vi "XYStage.TestLauncher.vi"() -> ()   [LabVIEW 2013]
doc: "JKI State Machine Objects (SMO) 1.0.0.5\nJKI - JKI\nCopyright (c) 2016, JKI"
uses:
  <vilib>/JKI/JKI SMO/SMO/SMO.lvclass
  XYStage.lvclass
  <vilib>/JKI/JKI SMO/SMO/Typedefs/SMOState --Enum.ctl
  Typedefs/(real)Coords--Cluster.ctl
  Typedefs/Configuration--Cluster.ctl
  XYStage.Simulated/XYStage.Simulated.lvclass
  Typedefs/(counts)Coords--Cluster.ctl
panel:
  in  "Home":bool
  out "Move Complete":bool
  out "Counts":T1
  in  "List Positions":bool
  in  "Move to Position":bool
  in  "Named Positions":i32(listbox)
  in  "Name":string
  in  "Store Position":bool
  out "Current Position":T2
  in  "MoveRel":bool
  in  "Coords":T2
  in  "MoveAbs":bool
  out "error out":errorcluster
  in  "Stop":bool
  # "XY Stage Test Launcher"
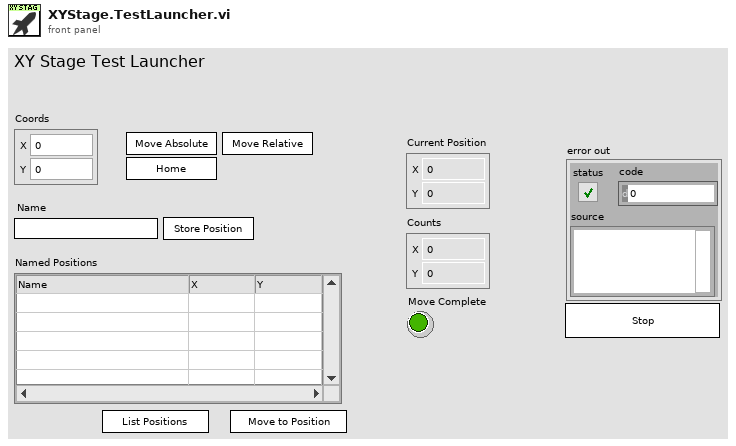
[diagram p1: front panel]
types:
  T1 = typedef "XYStage.lvclass/(counts)Coords--Cluster.ctl" = cluster{"X":i32, "Y":i32}
  T2 = typedef "XYStage.lvclass/(real)Coords--Cluster.ctl" = cluster{"X":dbl, "Y":dbl}
  T3 = typedef "XYStage.lvclass/Configuration--Cluster.ctl" = cluster{"Real-World Units":string, "Counts per Unit":dbl}
  T4 = typedef "SMO.lvclass/Public Events.ctl" = cluster{"Error":refnum<user-event>, "State":refnum<user-event>}
  T5 = typedef "XYStage.lvclass/PublicEvents--Cluster.ctl" = cluster{"MoveComplete":refnum<user-event>, "NewPosition":refnum<user-event>, "UpdatedNamedPosition":refnum<user-event>, "MoveStarted":refnum<user-event>}
  T6 = cluster{"Event Registration Refnum":refnum<event-registration>}
  T7 = typedef "SMO.lvclass/SMOState --Enum.ctl" = enum16{"unknown", "Created", "Started", "Stopped"}
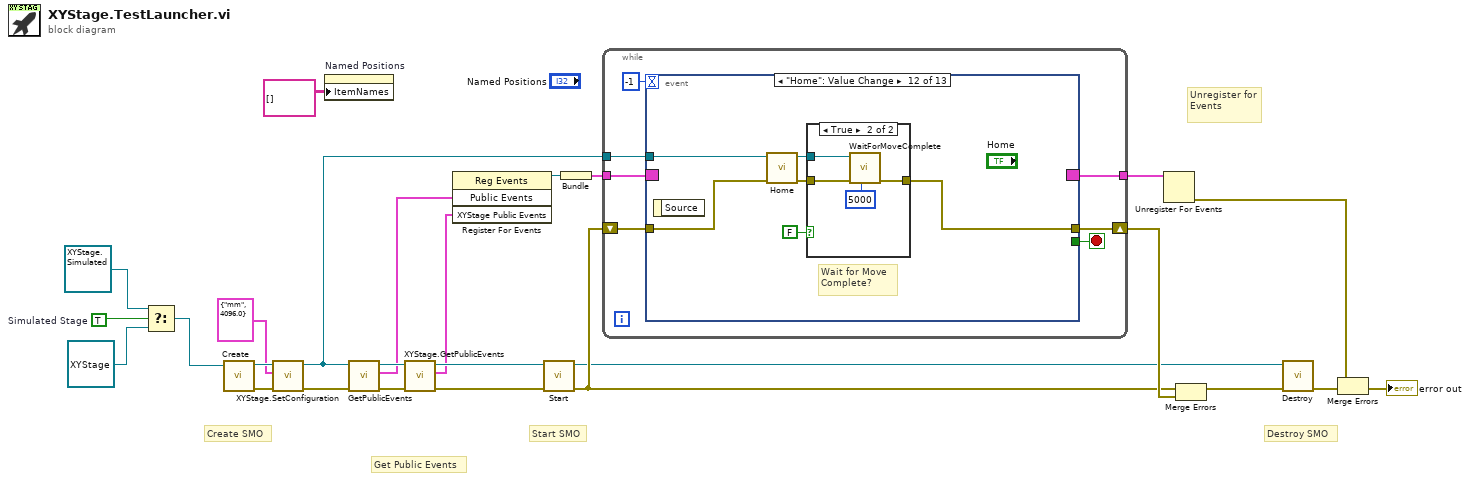
[diagram p0: block diagram]
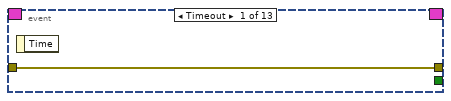
[diagram p2: hidden frame]
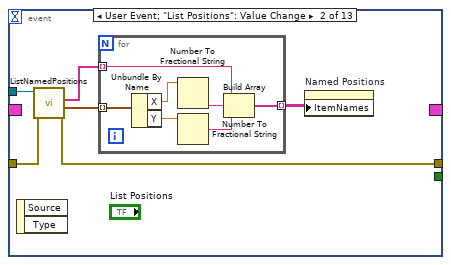
[diagram p3: hidden frame]
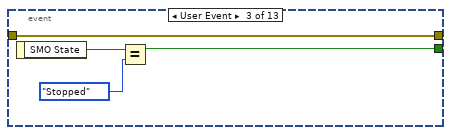
[diagram p4: hidden frame]
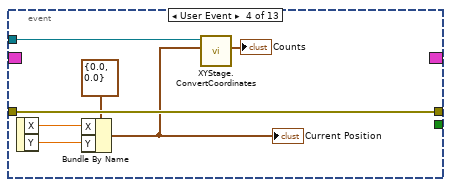
[diagram p5: hidden frame]
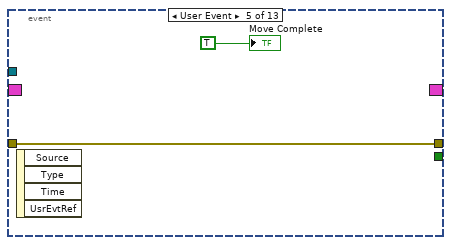
[diagram p6: hidden frame]
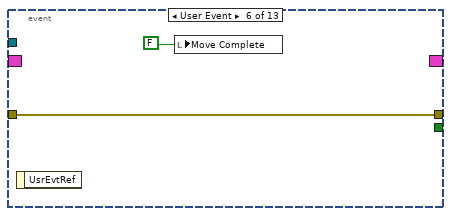
[diagram p7: hidden frame]
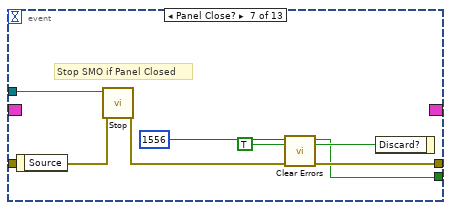
[diagram p8: hidden frame]
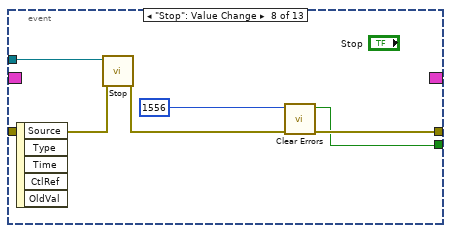
[diagram p9: hidden frame]
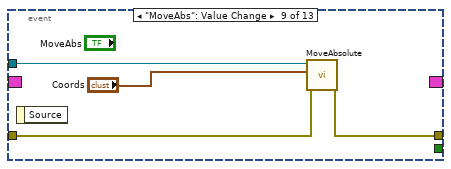
[diagram p10: hidden frame]
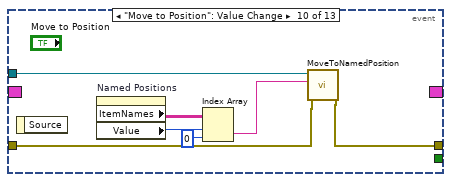
[diagram p11: hidden frame]
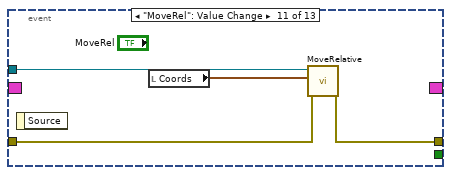
[diagram p12: hidden frame]
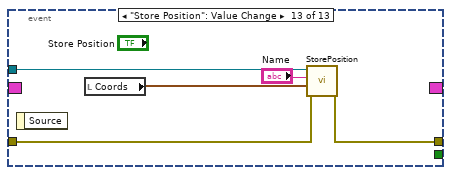
[diagram p14: hidden frame]
diagram:
  w4 = TRUE  # Simulated Stage
  # "Get Public Events"
  # "Start SMO"
  # "Destroy SMO"
  # "Create SMO"
  # "Unregister for Events"
  n1 = Select(t=refnum<class "XYStage.Simulated.lvclass"> refnum ("XYStage.Simulated.lvclass"), s=w4, f=refnum<class "XYStage.lvclass"> refnum ("SMO.Template.lvclass")) -> (s? t:f=w1:refnum<class "XYStage.lvclass">)
  n2 = call <vilib>:"Create.vi"("SMO"=w1) -> ("error out"=w10:errorcluster, "SMO out"=w8:refnum<class "XYStage.lvclass">)  [unwired: 8 in, 1 out]
  n3 = call "XYStage.SetConfiguration.vi"("error in (no error)"=w10, "Configuration"=T3 {"Real-World Units"="mm", "Counts per Unit"=4096.0}, "XYStage"=w8) -> ("error out"=w9:errorcluster, "XYStage out"=w7:refnum<class "XYStage.lvclass">)  [unwired: 7 in]
  n4 = property on="Named Positions" class="MCListbox (strict)"("ItemNames"=string[][] [] ("Item Names")) -> ()  [unwired: 2 in, 2 out]
  n5 = call <vilib>:"GetPublicEvents.vi"("error in (no error)"=w9, "SMO"=w7) -> ("error out"=w12:errorcluster, "Public Events"=w11:T4, "SMO out"=w13:refnum<class "XYStage.lvclass">)  [unwired: 7 in]
  n6 = call "XYStage.GetPublicEvents.vi"("error in (no error)"=w12, "XYStage"=w13) -> ("error out"=w14:errorcluster, "XYStage Public Events"=w16:T5, "XYStage out"=w17:refnum<class "XYStage.lvclass">)  [unwired: 7 in]
  n7 = register-events(w11, w16) -> (reference out=w15:refnum<event-registration>)  [unwired: 2 in, 1 out]
  n8 = call <vilib>:"Start.vi"("error in (no error)"=w14, "SMO"=w17) -> ("error out"=w20:errorcluster, "SMO out"=w18:refnum<class "XYStage.lvclass">)  [unwired: 8 in]
  n9 = Bundle("Event Registration Refnum"=w15) -> (w25:T6)  [unwired: 1 in]
  n10 = while {
    shift-right: [w32] -> w24
    shift-left: w20 -> [w31]
    tunnel: w25 -> [w30]
    tunnel: [w29] -> w26
    tunnel: w7 -> [w28]
    stop <- w33 stop-if-true
    n11 = event shown="[11] \"Home\": Value Change" {
      selector: w30 -> [_ _ _ _ _ _ _ _ _ _ _ _ _]
      dyn-events: [_ _ _ _ _ _ _ _ _ _ _ _ _] -> w29
      timeout: -1 -> [_ _ _ _ _ _ _ _ _ _ _ _ _]
      tunnel: [_ _ w49 _ _ _ w64 w71 _ _ _ _ _] -> w33
      tunnel: w28 -> [_ w40 _ w54 _ _ w69 w75 w79 w86 w89 w96 w106]
      tunnel: [w34 w38 w51 w58 w60 w62 w65 w72 w77 w84 w87 w93 w103] -> w32
      tunnel: w31 -> [w34 w39 w51 w58 w60 w62 w68 w74 w78 w85 w88 w92 w104]
      event Timeout {
        n12 = event-data() -> ()  [unwired: 1 in, 1 out]
      }
      event User Event; "List Positions": Value Change {
        n13 = event-data() -> ()  [unwired: 1 in, 2 out]
        n14 = call "ListNamedPositions.vi"("error in (no error)"=w39, "XYStage"=w40) -> ("error out"=w38:errorcluster, "Positions"=w37:T2[], "Names"=w36:string[])  [unwired: 6 in, 1 out]
        n15 = for {
          tunnel: w37 -> [w47] mode=indexing
          tunnel: w36 -> [w44] mode=indexing
          tunnel: [w41] -> w35 mode=indexing
          n16 = Unbundle By Name(w47) -> ("X"=w46:dbl, "Y"=w45:dbl)
          n17 = Number To Fractional String(number=w46) -> (F-format string=w43:string)  [unwired: 3 in]
          n18 = Number To Fractional String(number=w45) -> (F-format string=w42:string)  [unwired: 3 in]
          n19 = Build Array(w44, w43, w42) -> (w41:string[])
        }
        n20 = property on="Named Positions" class="MCListbox (strict)"("ItemNames"=w35) -> ()  [unwired: 2 in, 2 out]
      }
      event User Event {
        n21 = event-data() -> ("SMO State"=w50:T7)  [unwired: 1 in]
        n22 = Equal?(x=w50, y=SMOState_--Enum."Stopped") -> (x = y?=w49:bool)
      }
      event User Event {
        n23 = event-data() -> ("X"=w56:dbl, "Y"=w55:dbl)  [unwired: 1 in]
        n24 = Bundle By Name(cluster=T2 {"X"=0.0, "Y"=0.0} ("Coords"), "X"=w56, "Y"=w55) -> (w53:T2)
        "Current Position" <- w53
        n25 = call-dynamic "XYStage.ConvertCoordinates.vi"("Real Units Coords"=w53, "XYStage in"=w54) -> ("Counts out"=→"Counts":T1)  [unwired: 6 in, 3 out]
      }
      event User Event {
        n26 = event-data() -> ()  [unwired: 1 in, 4 out]
        "Move Complete" <- TRUE
      }
      event User Event {
        n27 = event-data() -> ()  [unwired: 1 in, 1 out]
        n28 = local write "Move Complete"(FALSE) -> ()
      }
      event Panel Close? {
        # "Stop SMO if Panel Closed"
        n29 = event-data() -> ()  [unwired: 1 in, 1 out]
        n30 = call <vilib>:"Stop.vi"("error in (no error)"=w68, "SMO"=w69) -> ("error out"=w66:errorcluster)  [unwired: 8 in, 1 out]
        n31 = call <vilib>:"Clear Errors.vi"("error in (no error)"=w66, "specific error code to clear (0: all)"=1556) -> ("error out"=w65:errorcluster, "specific error cleared?"=w64:bool)  [unwired: 4 in]
        n32 = event-data("Discard?"=TRUE ("OK")) -> ()  [unwired: 1 in, 1 out]
      }
      event "Stop": Value Change {
        n33 = event-data() -> ()  [unwired: 1 in, 5 out]
        n34 = call <vilib>:"Stop.vi"("error in (no error)"=w74, "SMO"=w75) -> ("error out"=w73:errorcluster)  [unwired: 8 in, 1 out]
        n35 = call <vilib>:"Clear Errors.vi"("error in (no error)"=w73, "specific error code to clear (0: all)"=1556) -> ("error out"=w72:errorcluster, "specific error cleared?"=w71:bool)  [unwired: 4 in]
      }
      event "MoveAbs": Value Change {
        n36 = event-data() -> ()  [unwired: 1 in, 1 out]
        n37 = call "MoveAbsolute.vi"("error in (no error)"=w78, "Units"="Coords", "XYStage"=w79) -> ("error out"=w77:errorcluster)  [unwired: 7 in, 1 out]
      }
      event "Move to Position": Value Change {
        n38 = event-data() -> ()  [unwired: 1 in, 1 out]
        n39 = property on="Named Positions" class="MCListbox (strict)"() -> ("ItemNames"=w83:string[][], "Value"=w82:i32)  [unwired: 2 in, 2 out]
        n40 = Index Array(array=w83, index (row)=w82, index (col)=0 ("disabled index (col)")) -> (element=w80:string)
        n41 = call "MoveToNamedPosition.vi"("error in (no error)"=w85, "MoveToNamedPosition"=w80, "XYStage"=w86) -> ("error out"=w84:errorcluster)  [unwired: 7 in, 1 out]
      }
      event "MoveRel": Value Change {
        n42 = event-data() -> ()  [unwired: 1 in, 1 out]
        n43 = local read "Coords"() -> (w90:T2)
        n44 = call "MoveRelative.vi"("error in (no error)"=w88, "Units"=w90, "XYStage"=w89) -> ("error out"=w87:errorcluster)  [unwired: 7 in, 1 out]
      }
      event "Home": Value Change {
        # "Wait for Move\nComplete?"
        n45 = event-data() -> ()  [unwired: 1 in, 1 out]
        n46 = call "Home.vi"("error in (no error)"=w92, "XYStage"=w96) -> ("error out"=w94:errorcluster, "XYStage out"=w95:refnum<class "XYStage.lvclass">)  [unwired: 8 in]
        n47 = case shown="True" FALSE {
          tunnel: w95 -> [_ w101]
          tunnel: w94 -> [w97 w100]
          tunnel: [w97 w99] -> w93
          frame False {
          }
          frame True {
            n48 = call "WaitForMoveComplete.vi"("timeout (5000 ms)"=5000, "error in (no error)"=w100, "XYStage"=w101) -> ("error out"=w99:errorcluster)  [unwired: 6 in, 2 out]
          }
        }
      }
      event "Store Position": Value Change {
        n49 = event-data() -> ()  [unwired: 1 in, 1 out]
        n50 = local read "Coords"() -> (w105:T2)
        n51 = call "StorePosition.vi"("error in (no error)"=w104, "Units"=w105, "Name"="Name", "XYStage"=w106) -> ("error out"=w103:errorcluster)  [unwired: 6 in, 1 out]
      }
    }
  }
  n52 = Unregister For Events(event registration refnum=w26) -> (error out=w23:errorcluster)  [unwired: 1 in]
  n53 = Merge Errors(w20, w24) -> (w19:errorcluster)
  n54 = call <vilib>:"Destroy.vi"("error in (no error)"=w19, "SMO"=w18) -> ("error out"=w21:errorcluster)  [unwired: 9 in]
  n55 = Merge Errors(w23, w21) -> (→"error out":errorcluster)
